vi "host-B.vi"() -> ()   [LabVIEW 2012]
uses:
  <vilib>/FPGAPlugInAG/PCI-7831R/niLvFpga_Open_PCI-7831R.vi
  <vilib>/Utility/error.llb/Error Cluster From Error Code.vi
  <vilib>/rvi/errors/niLvFpgaAdjustHostInterfaceError.vi
  <vilib>/FPGAPlugInAG/PCI-7831R/niLvFpga_Run_PCI-7831R.vi
  <vilib>/FPGAPlugInAG/PCI-7831R/niLvFpga_Abort_PCI-7831R.vi
  <vilib>/FPGAPlugInAG/PCI-7831R/niLvFpga_Close_PCI-7831R.vi
  <vilib>/rvi/interface/nirviOpenFPGA/nirviOpenFPGA.xnode
  SB130-XPS/Documents/FPGA-project-apporach-retraction/FPGA Bitfiles/Apporach-Retract_FPGATarget_LIAFPGA_OziXUy-ofuI.lvbitx
  LIA_FPGA.vi
  <vilib>/rvi/interface/nirviReadWriteControl/nirviReadWriteControl.xnode
  <vilib>/rvi/interface/nirviMethod/nirviMethod.xnode
  <vilib>/rvi/interface/nirviCloseFPGA/nirviCloseFPGA.xnode
  NiFpgaLv.dll
panel:
  out "3rd stages":i32
  out "3rd decimation":i32
  out "1st decimation":i32
  out "2nd decimation":i32
  in  "Time Constant [s]":dbl=1.0 min=0.0 step=0.0001 format="%.2f"
  in  "Filter Rolloff":enum16{"20 dB", "40 dB", "60 dB", "80 dB"}(ring)
  out "Actual Sampling Frequency":dbl
  in  "input range of 9205":dbl=10.0
  in  "Sampling Frequency":dbl=50000.0 min=1000.0 max=250000.0
  in  "stop":bool
  out "degree":dbl
  out "r":dbl(graph)
  out "y":dbl
  out "x":dbl
  out "f":dbl(graph)
  in  "dec2":i16=1
  in  "nominal freq":dbl=1000.0 min=500.0 max=125000.0
  in  "dec1":i16=1000
  in  "stages":i8=1 min=1 max=2
  in  "decimation":i16=1000
  # "Sampling Frequency"
  # "CIC First Decimation"
  # "CIC Second Decimation"
  # "MA Stages"
  # "MA Decimation"
  # "PLL Nominal Frequency"
  # "PLL Frequency Output"
  # "LIA Output"
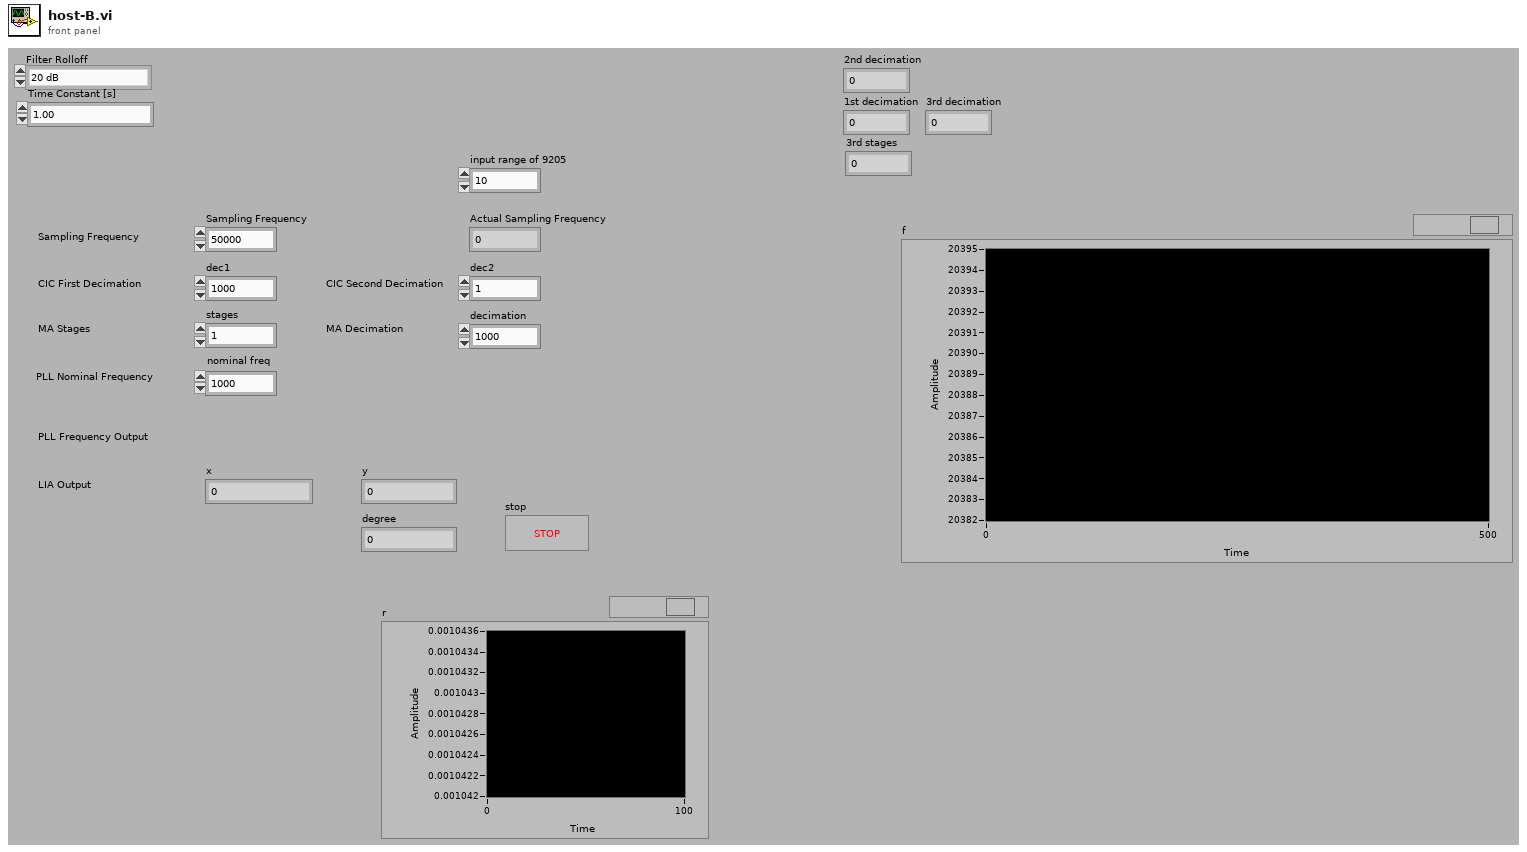
[diagram p1: front panel]
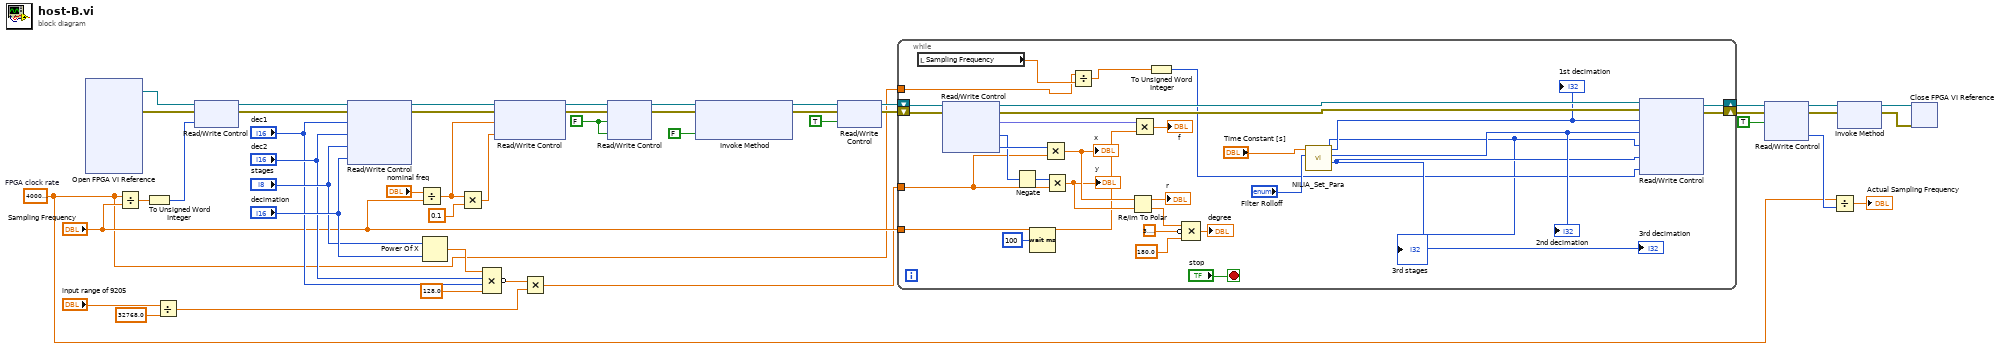
[diagram p0: block diagram]
diagram:
  w1 = 40000000.0  # FPGA clock rate
  w23 = FALSE ("start")
  n1 = xnode "Open FPGA VI Reference"() -> ("FPGA VI Reference Out"=w9:refnum<k20>, "error out"=w8:errorcluster)  [unwired: 2 in]
  n2 = Divide(x=w1, y="Sampling Frequency") -> (x/y=w16:dbl)
  n3 = To Unsigned Word Integer(number=w16) -> (unsigned 16bit integer=w15:u16)
  n4 = Divide(x="input range of 9205", y=32768.0) -> (x/y=w4:dbl)
  n5 = xnode "Read/Write Control"("FPGA VI Reference In"=w9, "error in"=w8, "Period"=w15) -> ("FPGA VI Reference Out"=w18:refnum<k20>, "error out"=w17:errorcluster)
  n6 = xnode "Read/Write Control"("FPGA VI Reference In"=w18, "error in"=w17, "dec1"="dec1", "dec2"="dec2", "stages"="stages", "decimation"="decimation") -> ("FPGA VI Reference Out"=w45:refnum<k20>, "error out"=w44:errorcluster)
  n7 = Divide(x="nominal freq", y="Sampling Frequency") -> (x/y=w12:dbl)
  n8 = Power Of X(1:"decimation", 2:"stages") -> (0:w40:dbl)
  n9 = Multiply(x=w12, y=0.1) -> (x*y=w10:dbl)
  n10 = Compound Arithmetic op=MULTIPLY(w40, "dec2", "dec1", 128.0) -> (invert w36:dbl)
  n11 = xnode "Read/Write Control"("FPGA VI Reference In"=w45, "error in"=w44, "nominal freq"=w12, "K"=w10) -> ("FPGA VI Reference Out"=w27:refnum<k20>, "error out"=w26:errorcluster)
  n12 = Multiply(x=w36, y=w4) -> (x*y=w5:dbl)
  n13 = xnode "Read/Write Control"("FPGA VI Reference In"=w27, "error in"=w26, "start"=w23, "stop"=w23) -> ("FPGA VI Reference Out"=w25:refnum<k20>, "error out"=w24:errorcluster)
  n14 = xnode "Invoke Method"("FPGA VI Reference In"=w25, "error in"=w24, "Wait Until Done (F)"=FALSE) -> ("FPGA VI Reference Out"=w32:refnum<k20>, "error out"=w30:errorcluster)
  n15 = xnode "Read/Write Control"("FPGA VI Reference In"=w32, "error in"=w30, "start"=TRUE) -> ("FPGA VI Reference Out"=w31:refnum<k20>, "error out"=w29:errorcluster)
  n16 = while {
    shift-right: [w57] -> w35
    shift-left: w31 -> [w75]
    shift-right: [w56] -> w34
    shift-left: w29 -> [w74]
    tunnel: w5 -> [w71]
    tunnel: "Sampling Frequency" -> [w60]
    tunnel: w1 -> [w49]
    stop <- "stop" stop-if-true
    n17 = local read "Sampling Frequency"() -> (w50:dbl)
    n18 = xnode "Read/Write Control"("FPGA VI Reference In"=w75, "error in"=w74) -> ("FPGA VI Reference Out"=w57:refnum<k20>, "error out"=w56:errorcluster, "f"=w61:fxp<+/-,32,0>, "channelQ"=w72:i64, "channelI"=w73:i64)
    n19 = Negate(x=w72) -> (-x=w58:i64)
    n20 = Wait (ms)(milliseconds to wait=u32 100) -> ()  [unwired: 1 out]
    n21 = Multiply(x=w73, y=w71) -> (x*y=w70:dbl)
    "x" <- w70
    n22 = Multiply(x=w58, y=w71) -> (x*y=w69:dbl)
    "y" <- w69
    n23 = Divide(x=w49, y=w50) -> (x/y=w48:dbl)
    n24 = Re/Im To Polar(2:w69, 3:w70) -> (0:w67:dbl, 1:→"r":dbl)
    n25 = Multiply(x=w61, y=w60) -> (x*y=→"f":dbl)
    n26 = To Unsigned Word Integer(number=w48) -> (unsigned 16bit integer=w47:u16)
    n27 = Compound Arithmetic op=MULTIPLY(w67, invert 3.141592653589793, 180.0 ("value")) -> (→"degree":dbl)
    n28 = call "NILIA_Set_Para.vi"("rolloff"="Filter Rolloff", "TC [sec]"="Time Constant [s]") -> ("3rd stages"=w46:i32, "3rd decimation"=w51:i32, "2nd decimation"=w52:i32, "1st decimation"=w53:i32)  [unwired: 5 in, 1 out]
    "2nd decimation" <- w52
    "1st decimation" <- w53
    "3rd decimation" <- w51
    "3rd stages" <- w46
    n29 = xnode "Read/Write Control"("FPGA VI Reference In"=w57, "error in"=w56, "dec1"=w53, "dec2"=w52, "stages"=w46, "decimation"=w51, "Period"=w47) -> ()  [unwired: 2 out]
  }
  n30 = xnode "Read/Write Control"("FPGA VI Reference In"=w35, "error in"=w34, "stop"=TRUE) -> ("FPGA VI Reference Out"=w22:refnum<k20>, "error out"=w21:errorcluster, "ticks"=w3:u16)
  n31 = Divide(x=w1, y=w3) -> (x/y=→"Actual Sampling Frequency":dbl)
  n32 = xnode "Invoke Method"("FPGA VI Reference In"=w22, "error in"=w21) -> ("FPGA VI Reference Out"=w20:refnum<k20>, "error out"=w19:errorcluster)
  n33 = xnode "Close FPGA VI Reference"("FPGA VI Reference In"=w20, "error in"=w19) -> ()  [unwired: 1 out]
